vi "getShootingAngle.vi"(0 "delta_y":dbl, 1 "initial_x":dbl, 2 "initial_z":dbl, 3 "final_x":dbl, 4 "final_z":dbl, 5 "initial_velocity_y":dbl, 6 "robot_velocity_x":dbl, 7 "robot_velocity_y":dbl) -> (14 "cowl_angle":dbl, 15 "turret_angle":dbl, 16 "firing_speed":dbl)   [LabVIEW 2019]
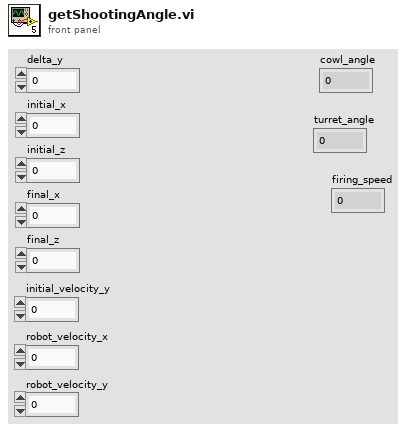
[diagram p1: front panel]
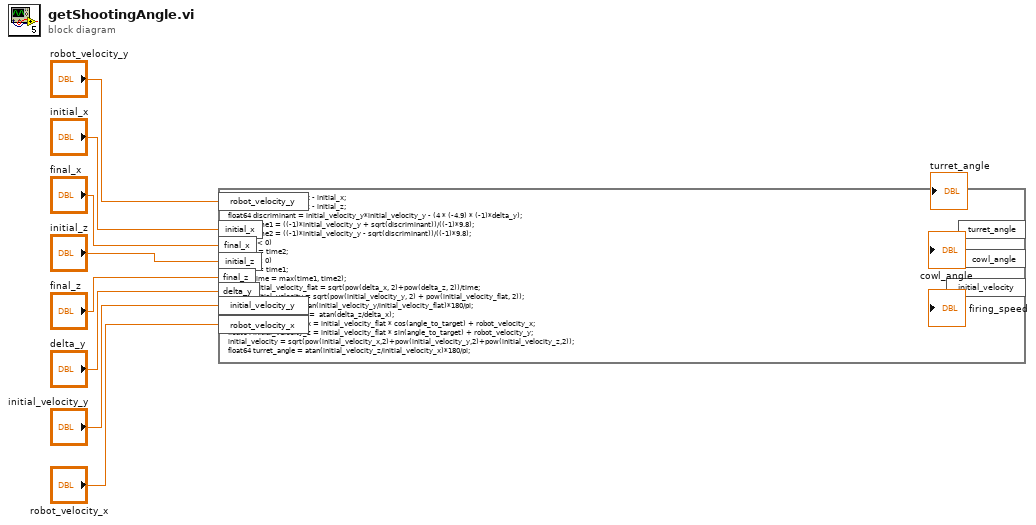
[diagram p0: block diagram]
diagram:
  n1 = formula code="float64 delta_x = final_x - initial_x;\nfloat64 delta_z = final_z - initial_z;\nfloat64 discriminant = initial_velocity_y*initial_velocity_y - (4 * (-4.9) * (-1)*delta_y);\nfloat64 time1 = ((-1)*initial_velocity_y + sqrt(discriminant))/((-1)*9.8);\nfloat64 time2 = ((-1)*initial_velocity_y - sqrt(discriminant))/((-1)*9.8);\nif(time1 < 0)\n    time1 = time2;\nif(time2 < 0)\n    time2 = time1;\nfloat64 time = max(time1, time2);\nfloat64 initial_velocity_flat = sqrt(pow(delta_x, 2)+pow(delta_z, 2))/time;\nfloat64 initial_velocity = sqrt(pow(initial_velocity_y, 2) + pow(initial_velocity_flat, 2));\nfloat64 cowl_angle = atan(initial_velocity_y/initial_velocity_flat)*180/pi;\nfloat64 angle_to_target =  atan(delta_z/delta_x);\nfloat64 initial_velocity_x = initial_velocity_flat * cos(angle_to_target) + robot_velocity_x;\nfloat64 initial_velocity_z = initial_velocity_flat * sin(angle_to_target) + robot_velocity_y;\ninitial_velocity = sqrt(pow(initial_velocity_x,2)+pow(initial_velocity_y,2)+pow(initial_velocity_z,2));\nfloat64 turret_angle = atan(initial_velocity_z/initial_velocity_x)*180/pi;"("initial_x"="initial_x", "final_x"="final_x", "initial_z"="initial_z", "final_z"="final_z", "delta_y"="delta_y", "initial_velocity_y"="initial_velocity_y", "robot_velocity_x"="robot_velocity_x", "robot_velocity_y"="robot_velocity_y") -> ("turret_angle"=→"turret_angle":dbl, "cowl_angle"=→"cowl_angle":dbl, "initial_velocity"=→"firing_speed":dbl)
